vi "SubVI_Arm_Setup.vi"(6 "Arm IP Address":string="192.168.10.16", 8 "error in (no error)":errorcluster, 11 "Arm Sampling Rate":u32) -> (0 "error out":errorcluster, 2 "Max Position":dbl, 3 "Arm TCP ID":refnum<k5>)   [LabVIEW 2020]
uses:
  Global 1.vi
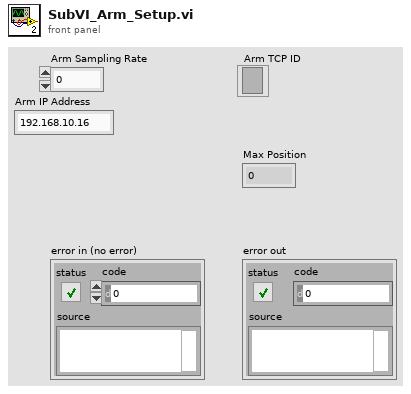
[diagram p1: front panel]
types:
  T1 = enum16{"Standard", "Buffered", "CRLF", "Immediate"}
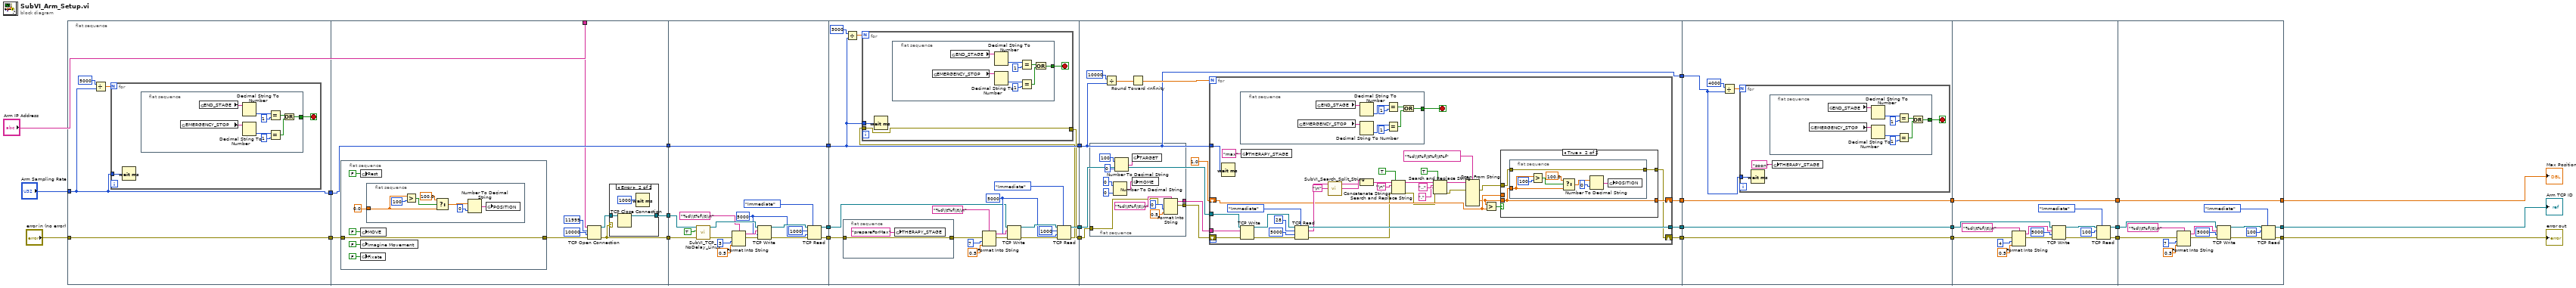
[diagram p0: block diagram]
diagram:
  n1 = flat-sequence {
    tunnel: [w29] -> w4
    tunnel: "error in (no error)" -> [w29]
    tunnel: "Arm Sampling Rate" -> [w28]
    tunnel: [w28] -> w3
    tunnel: [w44] -> w23
    tunnel: w4 -> [w49]
    tunnel: [w51] -> w22
    tunnel: [w50] -> w21
    tunnel: w3 -> [w44]
    tunnel: "Arm IP Address" -> [w43]
    tunnel: w23 -> [w69]
    tunnel: [w69] -> w20
    tunnel: w22 -> [w85]
    tunnel: w21 -> [w84]
    tunnel: [w74] -> w19
    tunnel: [w73] -> w18
    tunnel: w20 -> [w89]
    tunnel: [w89] -> w17
    tunnel: w19 -> [w95]
    tunnel: w18 -> [w93]
    tunnel: [w87] -> w16
    tunnel: [w94] -> w15
    tunnel: w17 -> [w122]
    tunnel: [w123] -> w10
    tunnel: w16 -> [w121]
    tunnel: w15 -> [w124]
    tunnel: [w126] -> w8
    tunnel: [w125] -> w6
    tunnel: [w122] -> w2
    tunnel: w10 -> [w205]
    tunnel: [w205] -> w9
    tunnel: w8 -> [w204]
    tunnel: [w204] -> w7
    tunnel: w6 -> [w203]
    tunnel: [w203] -> w5
    tunnel: w2 -> [w200]
    tunnel: w9 -> [w218]
    tunnel: [w218] -> w14
    tunnel: w7 -> [w221]
    tunnel: w5 -> [w220]
    tunnel: [w222] -> w13
    tunnel: [w219] -> w12
    tunnel: [w235] -> w27
    tunnel: [w234] -> w24
    tunnel: [w233] -> w26
    tunnel: w14 -> [w233]
    tunnel: w13 -> [w237]
    tunnel: w12 -> [w236]
    frame #0 {
      n2 = Divide(x=u32 5000 ("milliseconds to wait"), y=w28) -> (x/y=w30:dbl)
      n3 = for {
        N: w30 -> [_]
        tunnel: w28 -> [w33]
        stop <- w32 stop-if-true
        n4 = Wait (ms)(milliseconds to wait=w33) -> ()  [unwired: 1 out]
        n5 = flat-sequence {
          tunnel: [w34] -> w32
          frame #0 {
            n6 = global read "Global 1.vi" "EMERGENCY_STOP"() -> (w37:string)
            n7 = global read "Global 1.vi" "END_STAGE"() -> (w42:string)
            n8 = Decimal String To Number(string=w42) -> (number=w41:i32)  [unwired: 2 in, 1 out]
            n9 = Decimal String To Number(string=w37) -> (number=w39:i32)  [unwired: 2 in, 1 out]
            n10 = Equal?(x=w41, y=1) -> (x = y?=w35:bool)
            n11 = Equal?(x=w39, y=1) -> (x = y?=w36:bool)
            n12 = Or(x=w35, y=w36) -> (x .or. y?=w34:bool)
          }
        }
      }
    }
    frame #1 {
      n13 = flat-sequence {
        tunnel: w49 -> [w57]
        tunnel: [w57] -> w45
        frame #0 {
          n14 = global write "Global 1.vi" "Rest"(FALSE ("Rest")) -> ()
          n15 = global write "Global 1.vi" "MOVE"(FALSE ("MOVE")) -> ()
          n16 = global write "Global 1.vi" "Imagine Movement"(FALSE ("Imagine Movement")) -> ()
          n17 = global write "Global 1.vi" "Fixate"(FALSE ("Fixate")) -> ()
          n18 = flat-sequence {
            tunnel: 0.0 ("Arm_position") -> [w58]
            frame #0 {
              n19 = Greater?(x=w58, y=100) -> (0:w63:bool)
              n20 = Select(t=100.0, s=w63, f=w58) -> (s? t:f=w60:dbl)
              n21 = Number To Decimal String(number=w60, width (-)=i16 0) -> (decimal integer string=w59:string)
              n22 = global write "Global 1.vi" "POSITION"(w59) -> ()
            }
          }
        }
      }
      n23 = TCP Open Connection(address=w43, remote port or service name=11999, timeout ms (60000)=10000, error in (no error)=w45) -> (connection ID=w46:refnum<k5>, error out=w51:errorcluster)  [unwired: 1 in]
      n24 = case shown="Error" w51 {
        tunnel: [w65 w66] -> w50
        tunnel: w46 -> [w65 w67]
        frame No Error {
        }
        frame Error {
          n25 = TCP Close Connection(connection ID=w67) -> (connection ID out=w66:refnum<k5>)  [unwired: 2 in, 1 out]
          n26 = Wait (ms)(milliseconds to wait=1000) -> ()  [unwired: 1 out]
        }
      }
    }
    frame #2 {
      w70 = 5000 ("timeout ms (25000)")
      n27 = call "SubVI_TCP_NoDelay_Linux.vi"("error in (no error)"=w85, "TCP_NODELAY (true)"=TRUE, "connID"=w84) -> ("error out"=w78:errorcluster, "connID 2"=w83:refnum<k5>)  [unwired: 3 in]
      n28 = Format Into String(format string="%d\\t%f\\t\\n", error in=w78, 3 ("input 1"), 0.5) -> (resulting string=w79:string, error out=w77:errorcluster)  [unwired: 1 in]
      n29 = TCP Write(connection ID=w83, data in=w79, error in (no error)=w77, 9:w70) -> (connection ID out=w75:refnum<k5>, error out=w76:errorcluster)  [unwired: 1 out]
      n30 = TCP Read(connection ID=w75, bytes to read=1000, error in (no error)=w76, 7:T1."Immediate" ("mode (standard)"), 9:w70) -> (connection ID out=w74:refnum<k5>, error out=w73:errorcluster)  [unwired: 1 out]
    }
    frame #3 {
      w96 = 5000 ("timeout ms (25000)")
      n31 = flat-sequence {
        tunnel: w93 -> [w119]
        tunnel: [w119] -> w92
        frame #0 {
          n32 = global write "Global 1.vi" "THERAPY_STAGE"("prepareForMax" ("THERAPY_STAGE")) -> ()
        }
      }
      n33 = Divide(x=u32 3000 ("milliseconds to wait"), y=w89) -> (x/y=w90:dbl)
      n34 = Format Into String(format string="%d\\t%f\\t\\n", error in=w92, 7 ("input 1"), 0.5) -> (resulting string=w102:string, error out=w101:errorcluster)  [unwired: 1 in]
      n35 = TCP Write(connection ID=w95, data in=w102, error in (no error)=w101, 9:w96) -> (connection ID out=w99:refnum<k5>, error out=w100:errorcluster)  [unwired: 1 out]
      n36 = TCP Read(connection ID=w99, bytes to read=1000, error in (no error)=w100, 7:T1."Immediate" ("mode (standard)"), 9:w96) -> (connection ID out=w94:refnum<k5>, error out=w88:errorcluster)  [unwired: 1 out]
      n37 = for {
        N: w90 -> [_]
        tunnel: w89 -> [w108]
        tunnel: w88 -> [w106]
        tunnel: [w106] -> w87
        stop <- w107 stop-if-true
        n38 = Wait (ms)(milliseconds to wait=w108) -> ()  [unwired: 1 out]
        n39 = flat-sequence {
          tunnel: [w109] -> w107
          frame #0 {
            n40 = global read "Global 1.vi" "EMERGENCY_STOP"() -> (w112:string)
            n41 = global read "Global 1.vi" "END_STAGE"() -> (w117:string)
            n42 = Decimal String To Number(string=w117) -> (number=w116:i32)  [unwired: 2 in, 1 out]
            n43 = Decimal String To Number(string=w112) -> (number=w114:i32)  [unwired: 2 in, 1 out]
            n44 = Equal?(x=w116, y=1) -> (x = y?=w110:bool)
            n45 = Equal?(x=w114, y=1) -> (x = y?=w111:bool)
            n46 = Or(x=w110, y=w111) -> (x .or. y?=w109:bool)
          }
        }
      }
    }
    frame #4 {
      n47 = flat-sequence {
        tunnel: [w143] -> w129
        tunnel: w121 -> [w133]
        tunnel: [w132] -> w120
        frame #0 {
          n48 = Number To Decimal String(number=0, width (-)=i16 0) -> (decimal integer string=w138:string)
          n49 = Number To Decimal String(number=100, width (-)=i16 0) -> (decimal integer string=w135:string)
          n50 = global write "Global 1.vi" "HOME"(w138) -> ()
          n51 = global write "Global 1.vi" "TARGET"(w135) -> ()
          n52 = Format Into String(format string="%d\\t%f\\t\\n", error in=w133, 0 ("input 1"), 0.5) -> (resulting string=w143:string, error out=w132:errorcluster)  [unwired: 1 in]
        }
      }
      n53 = Divide(x=u32 10000 ("milliseconds to wait"), y=w122) -> (x/y=w130:dbl)
      n54 = Round Toward -Infinity(1:w130) -> (0:w131:dbl)
      n55 = for {
        N: w131 -> [_]
        shift-right: [w144] -> w126
        shift-left: w120 -> [w176]
        tunnel: w129 -> [w173]
        shift-right: [w152] -> w123
        shift-left: 1.0 -> [w161]
        tunnel: [w177] -> w125
        tunnel: w124 -> [w153]
        tunnel: w122 -> [w151]
        stop <- w149 stop-if-true
        n56 = Wait (ms)(milliseconds to wait=w151) -> ()  [unwired: 1 out]
        n57 = flat-sequence {
          tunnel: [w178] -> w149
          frame #0 {
            n58 = global read "Global 1.vi" "EMERGENCY_STOP"() -> (w181:string)
            n59 = global read "Global 1.vi" "END_STAGE"() -> (w186:string)
            n60 = Decimal String To Number(string=w186) -> (number=w185:i32)  [unwired: 2 in, 1 out]
            n61 = Decimal String To Number(string=w181) -> (number=w183:i32)  [unwired: 2 in, 1 out]
            n62 = Equal?(x=w185, y=1) -> (x = y?=w179:bool)
            n63 = Equal?(x=w183, y=1) -> (x = y?=w180:bool)
            n64 = Or(x=w179, y=w180) -> (x .or. y?=w178:bool)
          }
        }
        n65 = TCP Write(connection ID=w153, data in=w173, error in (no error)=w176) -> (connection ID out=w175:refnum<k5>, error out=w174:errorcluster)  [unwired: 1 in, 1 out]
        n66 = global write "Global 1.vi" "THERAPY_STAGE"("max" ("THERAPY_STAGE")) -> ()
        n67 = TCP Read(connection ID=w175, bytes to read=28, error in (no error)=w174, 7:T1."Immediate" ("mode (standard)"), 9:5000 ("timeout ms (25000)")) -> (connection ID out=w177:refnum<k5>, data out=w163:string, error out=w148:errorcluster)
        n68 = call <userlib>:"SubVI_Search_Split_String.vi"("search string/char (-)"="\n", "string"=w163) -> ("substring after match"=w168:string, "substring before match"=w167:string)  [unwired: 1 in, 1 out]
        n69 = Concatenate Strings(w168, w167) -> (w169:string)
        n70 = Search and Replace String(replace all?=TRUE ("replace all? (F)"), input string=w169, search string="\n", error in=w148) -> (result string=w159:string, error out=w147:errorcluster)  [unwired: 4 in, 2 out]
        n71 = Search and Replace String(replace all?=TRUE ("replace all? (F)"), input string=w159, search string="..", replace string="." ("replace string (\"\")"), error in=w147) -> (result string=w157:string, error out=w146:errorcluster)  [unwired: 3 in, 2 out]
        n72 = Scan From String(format string="%d\\t%f\\t%f\\t%f", input string=w157, error in=w146) -> (error out=w145:errorcluster, output 3=w154:dbl)  [unwired: 8 in, 2 out]
        n73 = Greater?(x=w154, y=w161) -> (0:w162:bool)
        n74 = case shown="True" w162 {
          tunnel: w154 -> [_ w191]
          tunnel: w161 -> [w188 _]
          tunnel: [w188 w191] -> w152
          tunnel: w145 -> [w187 w190]
          tunnel: [w187 w189] -> w144
          frame False {
          }
          frame True {
            n75 = flat-sequence {
              tunnel: w191 -> [w193]
              tunnel: w190 -> [w192]
              tunnel: [w192] -> w189
              frame #0 {
                n76 = Greater?(x=w193, y=100) -> (0:w198:bool)
                n77 = Select(t=100.0, s=w198, f=w193) -> (s? t:f=w195:dbl)
                n78 = Number To Decimal String(number=w195, width (-)=i16 0) -> (decimal integer string=w194:string)
                n79 = global write "Global 1.vi" "POSITION"(w194) -> ()
              }
            }
          }
        }
      }
    }
    frame #5 {
      n80 = Divide(x=u32 4000 ("milliseconds to wait"), y=w200) -> (x/y=w201:dbl)
      n81 = for {
        N: w201 -> [_]
        tunnel: w200 -> [w208]
        stop <- w206 stop-if-true
        n82 = Wait (ms)(milliseconds to wait=w208) -> ()  [unwired: 1 out]
        n83 = flat-sequence {
          tunnel: [w209] -> w206
          frame #0 {
            n84 = global read "Global 1.vi" "EMERGENCY_STOP"() -> (w212:string)
            n85 = global read "Global 1.vi" "END_STAGE"() -> (w217:string)
            n86 = Decimal String To Number(string=w217) -> (number=w216:i32)  [unwired: 2 in, 1 out]
            n87 = Decimal String To Number(string=w212) -> (number=w214:i32)  [unwired: 2 in, 1 out]
            n88 = Equal?(x=w216, y=1) -> (x = y?=w210:bool)
            n89 = Equal?(x=w214, y=1) -> (x = y?=w211:bool)
            n90 = Or(x=w210, y=w211) -> (x .or. y?=w209:bool)
          }
        }
        n91 = global write "Global 1.vi" "THERAPY_STAGE"("soon" ("THERAPY_STAGE")) -> ()
      }
    }
    frame #6 {
      n92 = Format Into String(format string="%d\\t%f\\t\\n", error in=w221, 4 ("input 1"), 0.5) -> (resulting string=w232:string, error out=w230:errorcluster)  [unwired: 1 in]
      n93 = TCP Write(connection ID=w220, data in=w232, error in (no error)=w230, 9:5000 ("timeout ms (25000)")) -> (connection ID out=w231:refnum<k5>, error out=w229:errorcluster)  [unwired: 1 out]
      n94 = TCP Read(connection ID=w231, bytes to read=100, error in (no error)=w229, 7:T1."Immediate" ("mode (standard)")) -> (connection ID out=w222:refnum<k5>, error out=w219:errorcluster)  [unwired: 1 in, 1 out]
    }
    frame #7 {
      n95 = Format Into String(format string="%d\\t%f\\t\\n", error in=w236, 7 ("input 1"), 0.5) -> (resulting string=w247:string, error out=w243:errorcluster)  [unwired: 1 in]
      n96 = TCP Write(connection ID=w237, data in=w247, error in (no error)=w243, 9:5000 ("timeout ms (25000)")) -> (connection ID out=w244:refnum<k5>, error out=w239:errorcluster)  [unwired: 1 out]
      n97 = TCP Read(connection ID=w244, bytes to read=100, error in (no error)=w239, 7:T1."Immediate" ("mode (standard)")) -> (connection ID out=w234:refnum<k5>, error out=w235:errorcluster)  [unwired: 1 in, 1 out]
    }
  }
  "error out" <- w27
  "Max Position" <- w26
  "Arm TCP ID" <- w24
